vi "Main.vi"(11 "Module Admin":refnum<class "Delacor_lib_QMH_Module Admin.lvclass">) -> ()   [LabVIEW 2020, in "Property Panel Launcher.lvlib"]
doc: "This template is based off of the Queued Message Handler design pattern and the Queued Message Handler project template that ships with LabVIEW.\n\nThe main difference is that the queue is private to this module and communication between modules is performed via Broadcast and Request events.\n\nRequest events are wrapped in public API methods and are handled in the Event Handling Loop (EHL) of this VI. Any module can register for Broadcast events sent by this module. The EHL generates messages based on user interface actions.\n\nThe Message Handling Loop (MHL) processes messages generated by the EHL, or by other messages. The messages are string values, so new messages can be added easily to the Message Cases case structure in the MHL. Each message cluster can also provide an optional value for Message Data, which is a variant that can be converted to whatever message-specific data is required.\n_____\nBased on Delacor QMH Project Template 5.0.0.82."
uses:
  Property Panel Launcher.lvlib
  <vilib>/Delacor/Delacor QMH/Libraries/Module Admin_class/Delacor_lib_QMH_Module Admin.lvclass
  Module Data--cluster.ctl
  <vilib>/Delacor/Delacor QMH/Libraries/Message Queue_class/Delacor_lib_QMH_Message Queue.lvclass/Delacor_lib_QMH_Message Queue.ctl
  Stop Argument--cluster.ctl
  <vilib>/Delacor/Delacor QMH/Libraries/Module Admin_class/Delacor_lib_QMH_Module Admin.lvclass/Delacor_lib_QMH_Module Admin.ctl
  Load Panel Argument--cluster.ctl
  <vilib>/Utility/miscctls.llb/LVPointTypeDef.ctl
  <vilib>/Delacor/Delacor QMH/Libraries/Message Queue_class/Delacor_lib_QMH_Enqueue Message (Single).vi
  <vilib>/Delacor/Delacor QMH/Libraries/Module Admin_class/Delacor_lib_QMH_Get External Launch.vi
  <vilib>/Utility/error.llb/Error Cluster From Error Code.vi
  <vilib>/ErrorRing/Error Ring.xnode
  <vilib>/Delacor/Delacor QMH/Libraries/Message Queue_class/Delacor_lib_QMH_Message Queue.lvclass
  Disabled Property Panel/Disabled Property Panel.lvlib
  Control Property Tree/Control Property Tree.lvlib
panel:
  in  "Simulate MHL Error":bool
  in  "Simulate EHL Error":bool
  out "error out":errorcluster
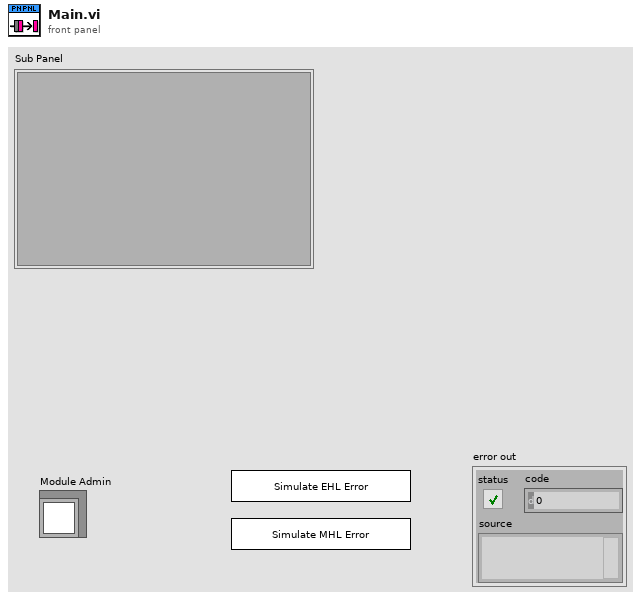
[diagram p1: front panel]
types:
  T1 = typedef "Property Panel Launcher.lvlib/Request Events--cluster.ctl" = cluster{"Stop Module":refnum<user-event>, "Show Panel":refnum<user-event>, "Hide Panel":refnum<user-event>, "Get Module Execution Status":refnum<user-event>, "Show Diagram":refnum<user-event>, "Load Panel":refnum<user-event>}
  T2 = typedef "Disabled Property Panel.lvlib/Broadcast Events--cluster.ctl" = cluster{"Module Did Init":refnum<user-event>, "Status Updated":refnum<user-event>, "Error Reported":refnum<user-event>, "Module Did Stop":refnum<user-event>, "Update Module Execution Status":refnum<user-event>, "Property Value Updated":refnum<user-event>}
  T3 = typedef "Property Panel Launcher.lvlib/Module Data--cluster.ctl" = cluster{"Status":string, "Current Selected Property":string}
  T4 = enum32{"invalid lock state", "Not Locked", "Locked (No Password)", "Password-protected"}
  T5 = typedef "Property Panel Launcher.lvlib/Stop Argument--cluster.ctl" = cluster{"Origin":string, "Exit via Stop Module Req?":bool, "Wait for Module to stop?":bool}
  T6 = typedef "Property Panel Launcher.lvlib/Load Panel Argument--cluster.ctl" = cluster{"New Selected Property":string}
  T7 = typedef "LVPointTypeDef.ctl" = cluster{"Horizontal":i16, "Vertical":i16}
  T8 = enum32{"Invalid", "Standard", "Closed", "Hidden", "Minimized", "Maximized"}
  T9 = cluster{"Property value":string, "Variant data":variant}
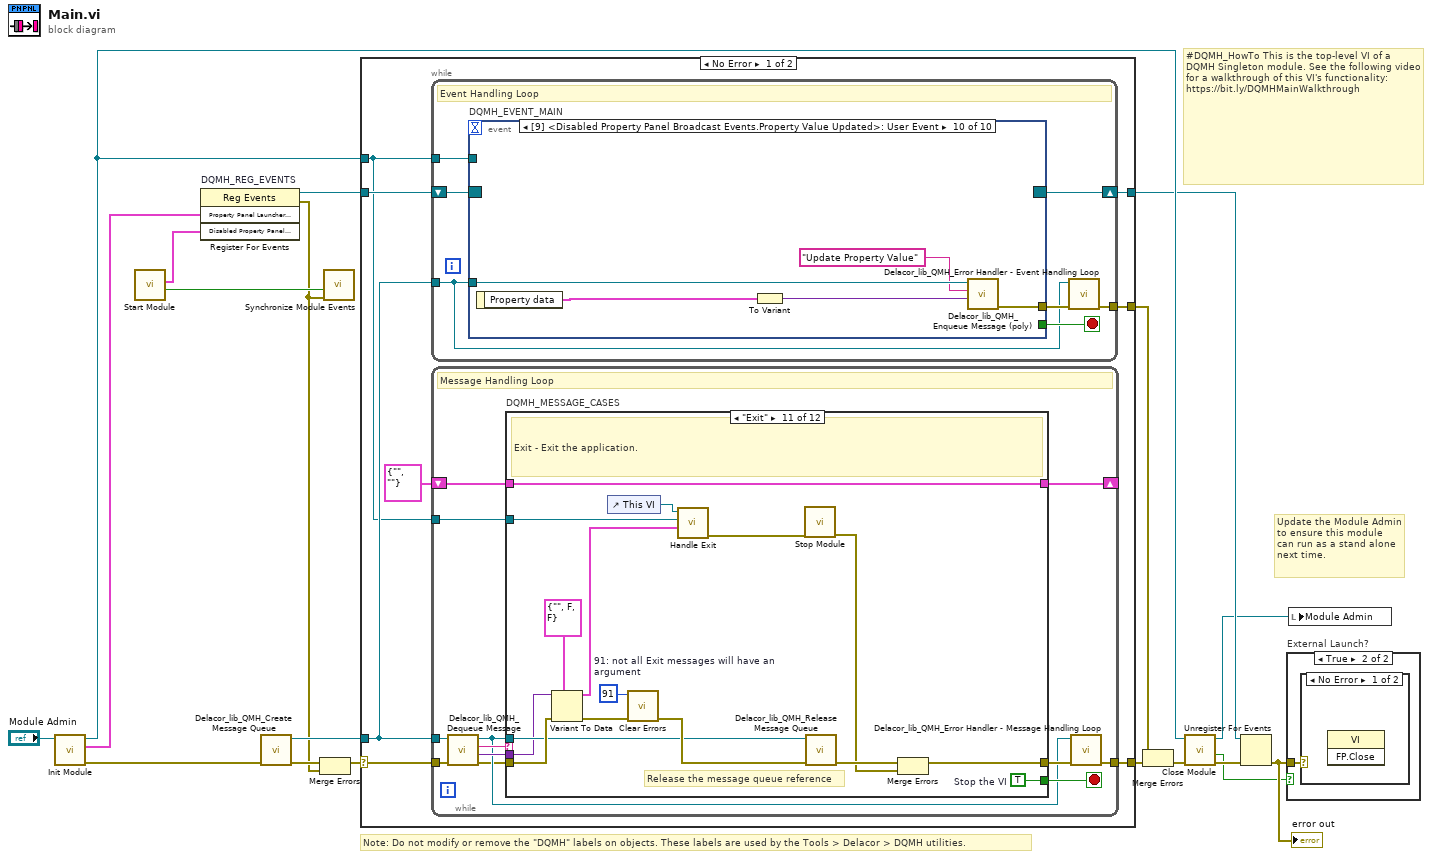
[diagram p0: block diagram]
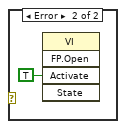
[diagram p3: hidden frame]
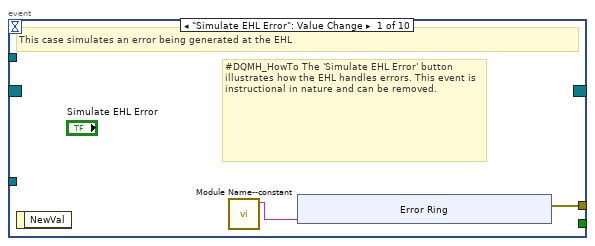
[diagram p4: hidden frame]
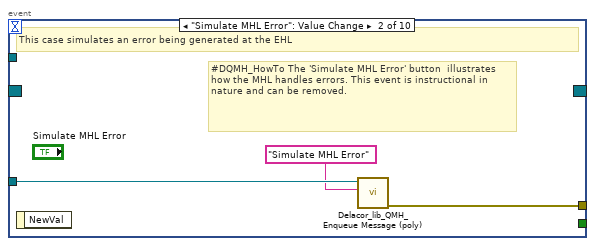
[diagram p5: hidden frame]
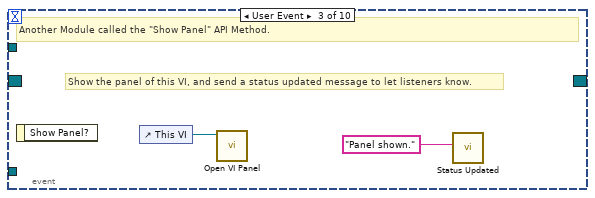
[diagram p6: hidden frame]
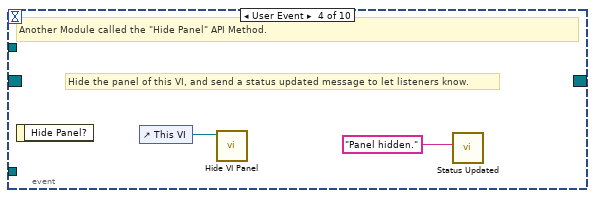
[diagram p7: hidden frame]
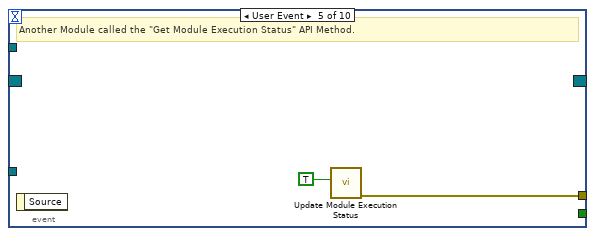
[diagram p8: hidden frame]
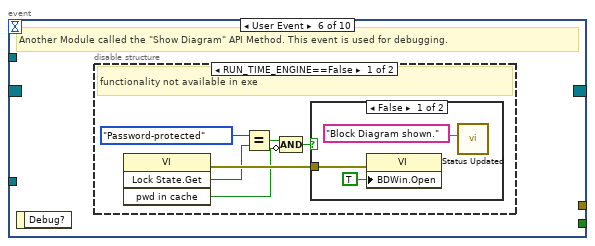
[diagram p9: hidden frame]
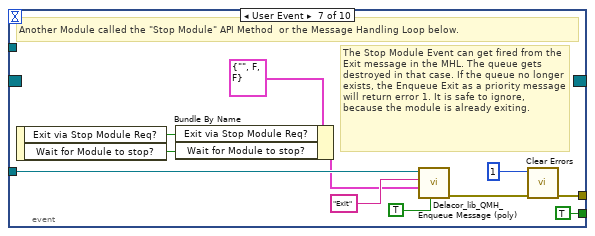
[diagram p12: hidden frame]
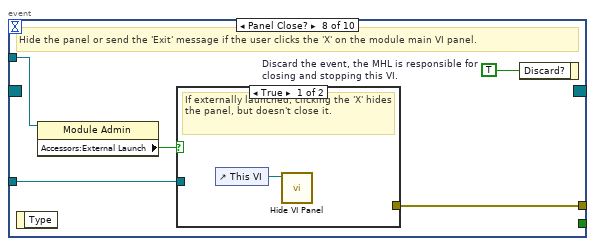
[diagram p13: hidden frame]
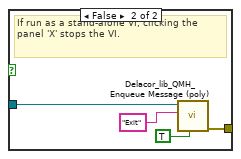
[diagram p14: hidden frame]
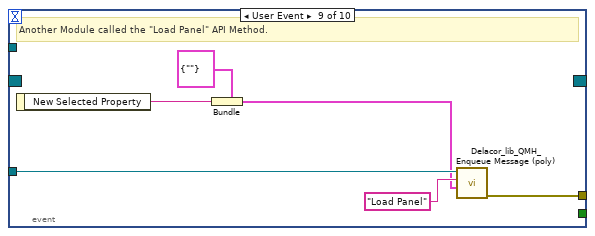
[diagram p15: hidden frame]
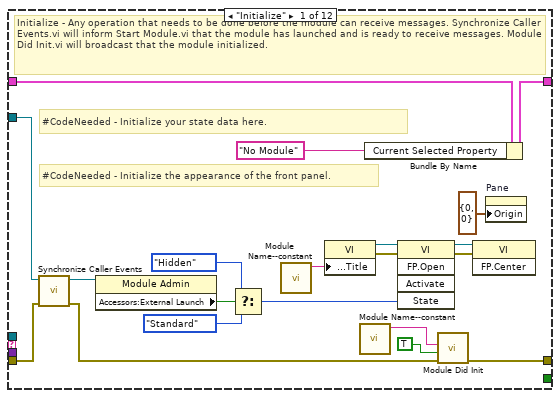
[diagram p16: hidden frame]
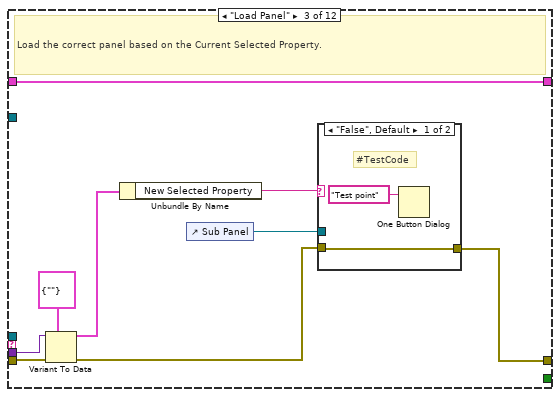
[diagram p18: hidden frame]
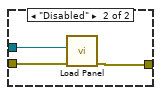
[diagram p19: hidden frame]
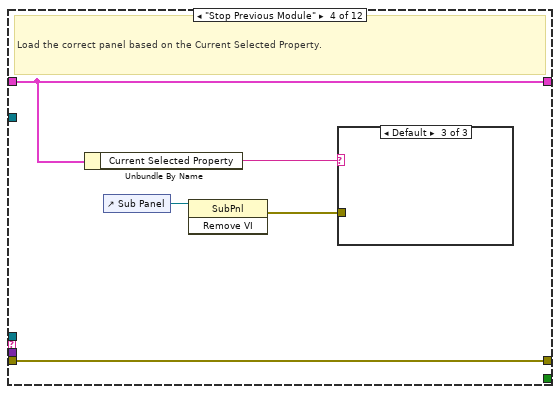
[diagram p20: hidden frame]
diagram:
  # "#DQMH_HowTo This is the top-level VI of a DQMH Singleton module. See the following video for a walkthrough of this VI's functionality: https://bit.ly/DQMHMainWalkthrough"
  # "Note: Do not modify or remove the \"DQMH\" labels on objects. These labels are used by the Tools > Delacor > DQMH utilities."
  # "Update the Module Admin to ensure this module can run as a stand alone next time."
  n1 = call "Init Module.vi"("Singleton Module Admin in"="Module Admin") -> ("error out"=w18:errorcluster, "Property Panel Launcher Request Events"=w8:T1, "Singleton Module Admin out"=w11:refnum<class "Delacor_lib_QMH_Module Admin.lvclass">)  [unwired: 8 in]
  n2 = call "Start Module.vi"() -> ("Wait for Event Sync?"=w3:bool, "Disabled Property Panel Broadcast Events"=w2:T2)  [unwired: 8 in, 2 out]
  n3 = register-events "DQMH_REG_EVENTS"(w8, w2) -> (reference out=w9:refnum<event-registration>, error out=w1:errorcluster)  [unwired: 2 in]
  n4 = call <vilib>:"Delacor_lib_QMH_Create Message Queue.vi"("error in (no error)"=w18) -> ("error out"=w13:errorcluster, "Message Queue"=w7:refnum<class "Delacor_lib_QMH_Message Queue.lvclass">)  [unwired: 9 in]
  n5 = Merge Errors(w13, w1) -> (w12:errorcluster)
  n6 = call "Synchronize Module Events.vi"("error in (no error)"=w1, "Wait for Event Sync?"=w3) -> ()  [unwired: 9 in, 1 out]
  n7 = case shown="No Error" w12 {
    selector: w12 -> [w25 w231]
    tunnel: [w27 w230] -> w19
    tunnel: [w24 w236] -> w10
    tunnel: w9 -> [w22 w236]
    tunnel: w7 -> [w21 w229]
    tunnel: [w26 _] -> w16
    tunnel: w11 -> [w20 w232]
    frame No Error {
      n8 = while {
        tunnel: w21 -> [w28]
        shift-right: [w31] -> w24
        shift-left: w22 -> [w32]
        tunnel: [w33] -> w26
        tunnel: w20 -> [w29]
        stop <- w30 stop-if-true
        # "Event Handling Loop"
        n9 = event "DQMH_EVENT_MAIN" shown="[9] <Disabled Property Panel Broadcast Events.Property Value Updated>: User Event" {
          selector: w32 -> [_ _ _ _ _ _ _ _ _ _]
          dyn-events: [_ _ _ _ _ _ _ _ _ _] -> w31
          timeout: _ -> [_ _ _ _ _ _ _ _ _ _]
          tunnel: [_ _ _ _ _ _ TRUE ("Discard?") _ _ _] -> w30
          tunnel: w28 -> [_ w45 _ _ _ _ w68 w75 w88 w92]
          tunnel: [w36 w46 _ _ w52 _ w71 w77 w83 w93] -> w34
          tunnel: w29 -> [_ _ _ _ _ _ _ w74 _ _]
          event "Simulate EHL Error": Value Change {
            # "#DQMH_HowTo The 'Simulate EHL Error' button  illustrates how the EHL handles errors. This event is instructional in nature and can be removed."
            # "This case simulates an error being generated at the EHL"
            n10 = event-data() -> ()  [unwired: 1 in, 1 out]
            n11 = call "Module Name--constant.vi"() -> ("Module Name"=w35:string)  [unwired: 11 in]
            n12 = xnode "Error Ring"("parameter 0"=w35) -> ("error out"=w36:errorcluster)
          }
          event "Simulate MHL Error": Value Change {
            # "#DQMH_HowTo The 'Simulate MHL Error' button  illustrates how the MHL handles errors. This event is instructional in nature and can be removed."
            # "This case simulates an error being generated at the EHL"
            n13 = event-data() -> ()  [unwired: 1 in, 1 out]
            n14 = call-poly <vilib>:"Delacor_lib_QMH_Enqueue Message (poly).vi"("Message"="Simulate MHL Error", "Message Queue in"=w45) -> ("error out"=w46:errorcluster)  [unwired: 8 in, 1 out]
          }
          event User Event {
            # "Show the panel of this VI, and send a status updated message to let listeners know."
            # "Another Module called the \"Show Panel\" API Method."
            n15 = event-data() -> ()  [unwired: 1 in, 1 out]
            n16 = control-ref of="This VI"() -> (w48:refnum<vi>)
            n17 = call "Open VI Panel.vi"("VI"=w48) -> ()  [unwired: 10 in, 1 out]
            n18 = call "Status Updated.vi"("Status"="Panel shown." ("format string")) -> ()  [unwired: 10 in, 1 out]
          }
          event User Event {
            # "Hide the panel of this VI, and send a status updated message to let listeners know."
            # "Another Module called the \"Hide Panel\" API Method."
            n19 = event-data() -> ()  [unwired: 1 in, 1 out]
            n20 = control-ref of="This VI"() -> (w50:refnum<vi>)
            n21 = call "Hide VI Panel.vi"("VI"=w50) -> ()  [unwired: 10 in, 1 out]
            n22 = call "Status Updated.vi"("Status"="Panel hidden." ("format string")) -> ()  [unwired: 10 in, 1 out]
          }
          event User Event {
            # "Another Module called the \"Get Module Execution Status\" API Method."
            n23 = event-data() -> ()  [unwired: 1 in, 1 out]
            n24 = call "Update Module Execution Status.vi"("Running?"=TRUE) -> ("error out"=w52:errorcluster)  [unwired: 10 in]
          }
          event User Event {
            # "Another Module called the \"Show Diagram\" API Method. This event is used for debugging."
            n25 = event-data() -> ()  [unwired: 1 in, 1 out]
            n26 = disable-structure shown="RUN_TIME_ENGINE==False" {
              frame condition #0 (active) {
                # "functionality not available in exe"
                n27 = invoke class="VI" method="Lock State.Get"() -> (error out=w58:errorcluster, "Get Lock State"=w57:T4, "pwd in cache"=w54:bool)  [unwired: 4 in, 1 out]
                n28 = Equal?(x=T4."Password-protected", y=w57) -> (x = y?=w55:bool)
                n29 = Compound Arithmetic op=AND(w55, invert w54) -> (w53:bool)
                n30 = case shown="False" w53 {
                  tunnel: w58 -> [w61 _]
                  frame False {
                    n31 = property class="VI"(error in=w61, "BDWin.Open"=TRUE ("Block Diagram Window:Open")) -> ()  [unwired: 1 in, 2 out]
                    n32 = call "Status Updated.vi"("Status"="Block Diagram shown." ("format string")) -> ()  [unwired: 10 in, 1 out]
                  }
                  frame True {
                    # "Password-protected VI, and the password is not in the cache. Do not show the diagram."
                  }
                }
              }
              frame condition #1 {
              }
            }
          }
          event User Event {
            # "The Stop Module Event can get fired from the Exit message in the MHL. The queue gets destroyed in that case. If the queue no longer exists, the Enqueue Exit as a priority message will return error 1. It is safe to ignore, because the module is already exiting."
            # "Another Module called the \"Stop Module\" API Method  or the Message Handling Loop below."
            n33 = event-data() -> ("Exit via Stop Module Req?"=w64:bool, "Wait for Module to stop?"=w63:bool)  [unwired: 1 in]
            n34 = Bundle By Name(cluster=T5 {"Origin"="", "Exit via Stop Module Req?"=FALSE, "Wait for Module to stop?"=FALSE} ("Stop Argument"), "Exit via Stop Module Req?"=w64, "Wait for Module to stop?"=w63) -> (w62:T5)
            n35 = call-poly <vilib>:"Delacor_lib_QMH_Enqueue Message (poly).vi"("Priority Message? (F)"=TRUE, "Message Data"=w62, "Message"="Exit", "Message Queue in"=w68) -> ("error out"=w72:errorcluster)  [unwired: 6 in, 1 out]
            n36 = call <vilib>:"Clear Errors.vi"("error in (no error)"=w72, "specific error code to clear (0: all)"=1) -> ("error out"=w71:errorcluster)  [unwired: 4 in, 1 out]
          }
          event Panel Close? {
            w76 = TRUE  # Discard the event, the MHL is responsible for closing and stopping this VI.
            # "Hide the panel or send the 'Exit' message if the user clicks the 'X' on the module main VI panel."
            n37 = event-data() -> ()  [unwired: 1 in, 1 out]
            n38 = property class="Module Admin"(reference=w74) -> ("Accessors:External Launch"=w73:bool)  [unwired: 1 in, 2 out]
            n39 = case shown="True" w73 {
              tunnel: w75 -> [_ w81]
              tunnel: [_ w82] -> w77
              frame True {
                # "If externally launched, clicking the 'X' hides the panel, but doesn't close it."
                n40 = control-ref of="This VI"() -> (w78:refnum<vi>)
                n41 = call "Hide VI Panel.vi"("VI"=w78) -> ()  [unwired: 10 in, 1 out]
              }
              frame False {
                # "If run as a stand-alone VI, clicking the panel 'X' stops the VI."
                n42 = call-poly <vilib>:"Delacor_lib_QMH_Enqueue Message (poly).vi"("Priority Message? (F)"=TRUE, "Message"="Exit", "Message Queue in"=w81) -> ("error out"=w82:errorcluster)  [unwired: 7 in, 1 out]
              }
            }
            n43 = event-data("Discard?"=w76) -> ()  [unwired: 1 in, 1 out]
          }
          event User Event {
            # "Another Module called the \"Load Panel\" API Method."
            n44 = event-data() -> ("New Selected Property"=w84:string)  [unwired: 1 in]
            n45 = Bundle(cluster=T6 {"New Selected Property"=""} ("Load Panel Argument"), "New Selected Property"=w84) -> (w85:T6)
            n46 = call-poly <vilib>:"Delacor_lib_QMH_Enqueue Message (poly).vi"("Message Data"=w85, "Message"="Load Panel", "Message Queue in"=w88) -> ("error out"=w83:errorcluster)  [unwired: 7 in, 1 out]
          }
          event User Event {
            n47 = event-data() -> ("Property data"=w90:T9)  [unwired: 1 in]
            n48 = To Variant(anything=w90) -> (Variant=w89:variant)
            n49 = call-poly <vilib>:"Delacor_lib_QMH_Enqueue Message (poly).vi"("Message Data"=w89, "Message"="Update Property Value", "Message Queue in"=w92) -> ("error out"=w93:errorcluster)  [unwired: 7 in, 1 out]
          }
        }
        n50 = call-dynamic "Delacor_lib_QMH_Error Handler - Event Handling Loop.vi"("error in (no error)"=w34, "Message Queue in"=w28) -> ("dup error in"=w33:errorcluster)  [unwired: 8 in, 1 out]
      }
      n51 = while {
        tunnel: w21 -> [w97]
        shift-right: [w101] -> _
        shift-left: T3 {"Status"="", "Current Selected Property"=""} ("Data Cluster") -> [w102]
        tunnel: w25 -> [w104]
        tunnel: [w103] -> w27
        tunnel: w20 -> [w95]
        stop <- w100 stop-if-true
        # "Message Handling Loop"
        n52 = call-dynamic "Delacor_lib_QMH_Dequeue Message.vi"("error in (no error)"=w104, "Message Queue in"=w97) -> ("error out"=w94:errorcluster, "Message Data"=w98:variant, "Message"=w99:string, "Message Queue out"=w96:refnum<class "Delacor_lib_QMH_Message Queue.lvclass">)  [unwired: 6 in]
        n53 = case "DQMH_MESSAGE_CASES" shown="\"Exit\"" w99 {
          selector: w99 -> [_ _ _ _ _ _ _ _ _ _ _ w216]
          tunnel: w96 -> [_ _ _ _ _ _ _ _ _ w185 w209 _]
          tunnel: w94 -> [w123 w127 w135 w144 w155 w163 w167 w169 w174 w192 w214 w218]
          tunnel: [w121 w127 w128 w144 w154 w157 w166 w169 w173 w188 w211 w219] -> w105
          tunnel: w102 -> [w112 w126 w134 w146 w148 w164 w165 w168 w171 w187 w201 w217]
          tunnel: [w111 w126 w134 w146 w150 w164 w165 w168 w171 w187 w201 w217] -> w101
          tunnel: [_ _ _ _ _ _ _ _ _ _ w208 _] -> w100
          tunnel: w98 -> [_ _ w132 _ w153 w162 _ _ _ w186 w207 _]
          tunnel: w95 -> [w113 _ _ _ _ _ _ _ _ w184 w202 _]
          frame "Initialize" {
            # "#CodeNeeded - Initialize the appearance of the front panel."
            # "#CodeNeeded - Initialize your state data here."
            # "Initialize - Any operation that needs to be done before the module can receive messages. Synchronize Caller Events.vi will inform Start Module.vi that the module has launched and is ready to receive messages. Module Did Init.vi will broadcast that the module initialized."
            n54 = call "Synchronize Caller Events.vi"("error in (no error)"=w123, "Singleton Module Admin in"=w113) -> ("error out"=w122:errorcluster, "Singleton Module Admin out"=w108:refnum<class "Delacor_lib_QMH_Module Admin.lvclass">)  [unwired: 8 in]
            n55 = property class="Module Admin"(reference=w108) -> ("Accessors:External Launch"=w117:bool)  [unwired: 1 in, 2 out]
            n56 = Select(t=T8."Hidden" ("State"), s=w117, f=T8."Standard" ("State")) -> (s? t:f=w114:T8)
            n57 = call "Module Name--constant.vi"() -> ("Module Name"=w120:string)  [unwired: 11 in]
            n58 = property class="VI"("Front Panel.Title"=w120) -> (reference out=w119:refnum<vi>, error out=w125:errorcluster)  [unwired: 2 in]
            n59 = call "Module Name--constant.vi"() -> ("Module Name"=w109:string)  [unwired: 11 in]
            n60 = Bundle By Name(cluster=w112, "Current Selected Property"="No Module" ("Initial Message")) -> (w111:T3)
            n61 = invoke class="VI" method="FP.Open"(reference=w119, error in=w125, "State"=w114) -> (reference out=w118:refnum<vi>, error out=w124:errorcluster)  [unwired: 2 in, 3 out]
            n62 = call "Module Did Init.vi"("error in (no error)"=w122, "Initialized?"=TRUE, "Origin"=w109) -> ("error out"=w121:errorcluster)  [unwired: 8 in]
            n63 = invoke class="VI" method="FP.Center"(reference=w118, error in=w124) -> ()  [unwired: 1 in, 3 out]
            n64 = property on="Pane" class="Pane"("Origin"=T7 {"Horizontal"=0, "Vertical"=0}) -> ()  [unwired: 2 in, 2 out]
          }
          frame "--- Module Specific ---" {
            # "Separator -- The following cases handle messages specific to this Module."
          }
          frame "Load Panel" {
            # "Load the correct panel based on the Current Selected Property."
            n65 = Variant To Data(error in=w135, type=T6 {"New Selected Property"=""} ("Load Panel Argument"), Variant=w132) -> (data=w133:T6, error out=w129:errorcluster)
            n66 = Unbundle By Name(w133) -> ("New Selected Property"=w131:string)
            n67 = control-ref of="Sub Panel"() -> (w130:refnum<vi>)
            n68 = case shown="\"False\", Default" w131 {
              tunnel: w130 -> [_ w141]
              tunnel: w129 -> [w138 w140]
              tunnel: [w138 w139] -> w128
              frame "False", Default {
                # "#TestCode"
                n69 = One Button Dialog(message="Test point") -> ()  [unwired: 1 in, 1 out]
              }
              frame "Disabled" {
                n70 = call "Load Panel.vi"("error in (no error)"=w140, "SubPnl Refnum"=w141) -> ("error out"=w139:errorcluster)  [unwired: 9 in]
              }
            }
          }
          frame "Stop Previous Module" {
            # "Load the correct panel based on the Current Selected Property."
            n71 = Unbundle By Name(w146) -> ("Current Selected Property"=w145:string)
            n72 = control-ref of="Sub Panel"() -> (w143:refnum<vi>)
            n73 = invoke class="SubPnl" method="Remove VI"(reference=w143) -> (error out=w142:errorcluster)  [unwired: 2 in, 2 out]
            n74 = case shown="Default" w145 {
              tunnel: w142 -> [w147 _ _]
              frame "Disabled" {
                n75 = call "Stop Module.vi"("error in (no error)"=w147) -> ()  [unwired: 10 in, 1 out]
              }
              frame "No Module" {
              }
              frame Default {
              }
            }
          }
          frame "Start New Module" {
            # "Load the correct panel based on the Current Selected Property."
            n76 = Variant To Data(error in=w155, type=T6 {"New Selected Property"=""} ("Load Panel Argument"), Variant=w153) -> (data=w151:T6, error out=w154:errorcluster)
            n77 = Unbundle By Name(w151) -> ("New Selected Property"=w149:string)
            n78 = Bundle By Name(cluster=w148, "Current Selected Property"=w149) -> (w150:T3)
          }
          frame "Update Property Value" {
            n79 = Variant To Data(error in=w163, type=T9 {"Property value"="", "Variant data"=variant} ("Property data"), Variant=w162) -> (data=w159:T9, error out=w156:errorcluster)
            n80 = Unbundle By Name(w159) -> ("Property value"=w161:string)
            n81 = call "Status Updated.vi"("error in (no error)"=w156, "Status"=w161) -> ("error out"=w158:errorcluster)  [unwired: 9 in]
            n82 = call "Update Property Value.vi"("error in (no error)"=w158, "Property data"=w159) -> ("error out"=w157:errorcluster)  [unwired: 9 in]
          }
          frame "---Copy This Frame---" {
            # "Duplicate this frame when creating new messages.  Change this comment in the duplicated frame to describe this message."
            n83 = Merge Errors(w167) -> (w166:errorcluster)
          }
          frame "--- Exit and Error Handling---" {
            # "Separator - The following cases handle errors and exit messages."
          }
          frame "Simulate MHL Error" {
            # "#DQMH_HowTo The 'Simulate MHL Error' button  illustrates how the MHL handles errors. This event is instructional in nature and can be removed."
            # "Simulate an error occurring at the MHL"
            n84 = call "Module Name--constant.vi"() -> ("Module Name"=w170:string)  [unwired: 11 in]
            n85 = xnode "Error Ring"("parameter 0"=w170) -> ("error out"=w172:errorcluster)
            n86 = Merge Errors(w174, w172) -> (w173:errorcluster)
          }
          frame "Error" {
            # "#CodeRecommended - If you ever change the name of this \"Error\" message, you'll need to update the name in the Check Loop Error.vi as well."
            # "#CodeRecommended - If the module is running in standalone mode (External Launch = FALSE), this code will pop up an error dialog and call the 'Exit' message if an error occurs. Add more fine-grained error handling here."
            # "Error - Check the error message data and respond accordingly. This message is sent by the \"Error Handler\" VIs at the end of each loop in this application."
            n87 = property class="Module Admin"(reference=w184) -> ("Accessors:External Launch"=w183:bool)  [unwired: 1 in, 2 out]
            n88 = Variant To Data(error in=w192, type=errorcluster {"status"=FALSE, "code"=0, "source"=""} ("error constant"), Variant=w186) -> (data=w193:errorcluster, error out=w190:errorcluster)
            n89 = call "Module Name--constant.vi"() -> ("Module Name"=w182:string)  [unwired: 11 in]
            n90 = call "Error Reported.vi"("Additional Information"=w182, "Error"=w193) -> ()  [unwired: 9 in, 1 out]
            n91 = case shown="False" w183 {
              tunnel: [w198 _] -> w189
              tunnel: w185 -> [w196 _]
              tunnel: w193 -> [w197 _]
              frame False {
                # "If the module is running standalone, then pop up an error dialog and call the \"Exit\" message."
                n92 = call <vilib>:"Simple Error Handler.vi"("error in (no error)"=w197) -> ()  [unwired: 4 in, 5 out]
                n93 = call-poly <vilib>:"Delacor_lib_QMH_Enqueue Message (poly).vi"("Priority Message? (F)"=TRUE, "Message"="Exit", "Message Queue in"=w196) -> ("error out"=w198:errorcluster)  [unwired: 7 in, 1 out]
              }
              frame True {
                # "If the module was launched externally, calling the Error Reported broadcast VI is the only action performed by the \"Error\" message. The module's caller can then process the error appropriately."
              }
            }
            n94 = Merge Errors(w190, w189) -> (w188:errorcluster)
            n95 = local write "error out"(w188) -> ()
          }
          frame "Exit" {
            w206 = 91  # 91: not all Exit messages will have an argument
            w208 = TRUE  # Stop the VI
            # "Release the message queue reference"
            # "Exit - Exit the application."
            n96 = Variant To Data(error in=w214, type=T5 {"Origin"="", "Exit via Stop Module Req?"=FALSE, "Wait for Module to stop?"=FALSE} ("Stop Argument"), Variant=w207) -> (data=w204:T5, error out=w210:errorcluster)
            n97 = control-ref of="This VI"() -> (w203:refnum<vi>)
            n98 = call <vilib>:"Clear Errors.vi"("error in (no error)"=w210, "specific error code to clear (0: all)"=w206) -> ("error out"=w213:errorcluster)  [unwired: 4 in, 1 out]
            n99 = call "Handle Exit.vi"("Stop Argument"=w204, "Admin in"=w202, "VI reference"=w203) -> ("error out"=w200:errorcluster)  [unwired: 7 in, 1 out]
            n100 = call "Stop Module.vi"("error in (no error)"=w200) -> ("error out"=w199:errorcluster)  [unwired: 10 in]
            n101 = call-dynamic "Delacor_lib_QMH_Release Message Queue.vi"("error in (no error)"=w213, "Message Queue"=w209) -> ("error out"=w212:errorcluster)  [unwired: 9 in]
            n102 = Merge Errors(w212, w199) -> (w211:errorcluster)
          }
          frame Default {
            # "'Default' case only runs if there is a message that isn't defined in any of the other cases.  Output a programming error."
            n103 = call "Module Name--constant.vi"() -> ("Module Name"=w215:string)  [unwired: 11 in]
            n104 = xnode "Error Ring"("parameter 0"=w216, "parameter 1"=w215) -> ("error out"=w220:errorcluster)
            n105 = Merge Errors(w218, w220) -> (w219:errorcluster)
          }
        }
        n106 = call-dynamic "Delacor_lib_QMH_Error Handler - Message Handling Loop.vi"("error in (no error)"=w105, "Message Queue in"=w96) -> ("dup error in"=w103:errorcluster)  [unwired: 8 in, 1 out]
      }
    }
    frame Error {
      # "Synchronize Caller Events.vi will inform Start Module.vi that the module has launched and will let the code calling Start Module.vi register for broadcasts and would permit the caller receive the broadcast that an error occurred at launch time."
      n107 = call-dynamic "Delacor_lib_QMH_Release Message Queue.vi"("error in (no error)"=w231, "Message Queue"=w229) -> ("error out"=w230:errorcluster)  [unwired: 9 in]
      n108 = call "Synchronize Caller Events.vi"("Singleton Module Admin in"=w232) -> ("error out"=w237:errorcluster)  [unwired: 9 in, 1 out]
      n109 = call "Module Name--constant.vi"() -> ("Module Name"=w235:string)  [unwired: 11 in]
      n110 = Format Into String(format string="An error occurred during initialization. %s is no longer running.", w235) -> (resulting string=w233:string)  [unwired: 2 in, 1 out]
      n111 = Merge Errors(w230, w237) -> (w238:errorcluster)
      n112 = call "Error Reported.vi"("Additional Information"=w233, "Error"=w238) -> ()  [unwired: 9 in, 1 out]
    }
  }
  n113 = Merge Errors(w16, w19) -> (w15:errorcluster)
  n114 = call "Close Module.vi"("error in (no error)"=w15, "Module Admin in"=w11) -> ("error out"=w17:errorcluster, "External Launch"=w4:bool, "Module Admin out"=w5:refnum<class "Delacor_lib_QMH_Module Admin.lvclass">)  [unwired: 7 in]
  n115 = Unregister For Events(event registration refnum=w10, error in=w17) -> (error out=w14:errorcluster)
  "error out" <- w14
  n116 = case "External Launch?" shown="True" w4 {
    tunnel: w14 -> [_ w239]
    frame False {
    }
    frame True {
      n117 = case shown="No Error" w239 {
        frame No Error {
          n118 = invoke class="VI" method="FP.Close"() -> ()  [unwired: 3 in, 3 out]
        }
        frame Error {
          n119 = invoke class="VI" method="FP.Open"("Activate"=TRUE ("Activate?")) -> ()  [unwired: 4 in, 5 out]
        }
      }
    }
  }
  n120 = local write "Module Admin"(w5) -> ()
